vi "Configure Frequency Offset.vi"(0 "VISA resource name":refnum<visa-resource-name>, 1 "Multiplier (1)":i32=1, 3 "Divisor (1)":i32=1, 4 "Offset (0.0)":dbl format="%^.3g", 5 "error in (no error)":errorcluster, 6 "Channel (1)":i32=1, 7 "Start (300.0E+3)":dbl=300000.0 format="%^.1e", 9 "Stop (300.0E+3)":dbl=300000.0 format="%^.1g", 10 "External Frequency State (F: Disabled)":bool, 11 "Avoid Spurious (F: Off)":bool, 12 "Port (1)":i32=1, 13 "X Axis Frequency (0: Normal Frequency)":u16(ring) items=["Normal frequency", "Normal frequency + frequency of the external signal source", "Normal frequency - frequency of the external signal source", "Frequency of the external signal source - normal frequency", "Normal frequency", "Frequency for the source port for the specified measurement parameter", "Frequency for the receiver port for the specified measurement parameter"]) -> (14 "VISA resource name out":refnum<visa-resource-name>, 19 "error out":errorcluster)   [LabVIEW 2020, in "Agilent ENA Series.lvlib"]
doc: "Configures frequency offset parameters.\n\n<B>Note:</B>\nThis VI is not valid for E5061B/E5063A, E5080A and E5080B."
uses:
  <instrlib>/Agilent ENA Series/Agilent ENA Series.lvlib
panel:
  # "Note:\nThis VI is not supported by the E5061B/E5063A, E5080A and E5080B."
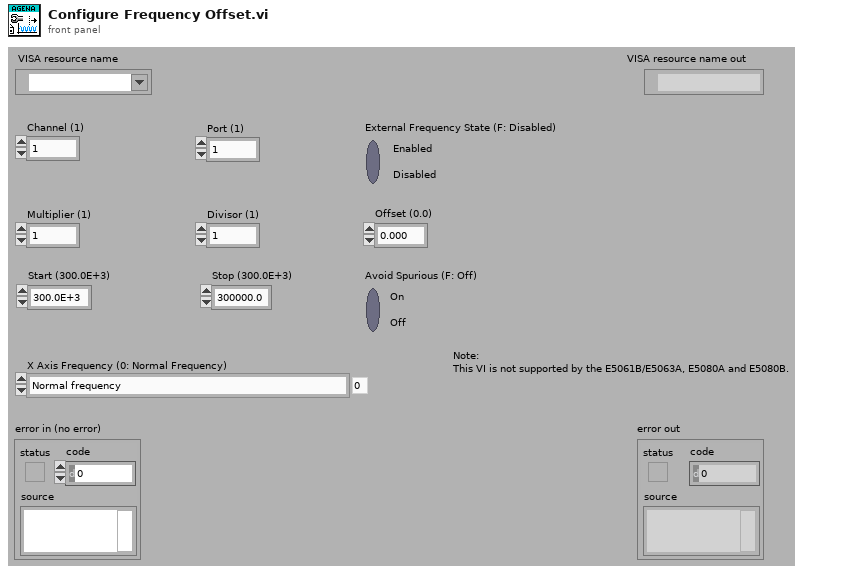
[diagram p1: front panel]
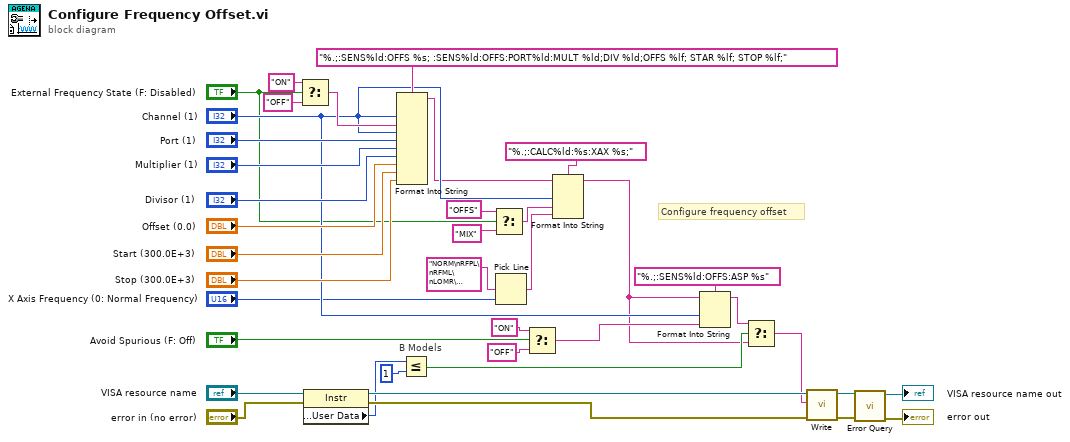
[diagram p0: block diagram]
diagram:
  # "Configure frequency offset"
  # "B Models"
  n1 = Select(t="ON", s="External Frequency State (F: Disabled)", f="OFF") -> (s? t:f=w36:string)
  n2 = property on="Property Node" class="Instr"(reference="VISA resource name", error in="error in (no error)") -> (reference out=w8:refnum<visa-resource-name>, error out=w7:errorcluster, "General Settings:User Data"=w5:u32)
  n3 = Format Into String(format string="%.;:SENS%ld:OFFS %s; :SENS%ld:OFFS:PORT%ld:MULT %ld;DIV %ld;OFFS %lf; STAR %lf; STOP %lf;", "Channel (1)", w36, "Channel (1)", "Port (1)", "Multiplier (1)", "Divisor (1)", "Offset (0.0)", "Start (300.0E+3)", "Stop (300.0E+3)") -> (resulting string=w2:string)  [unwired: 2 in, 1 out]
  n4 = Less Or Equal?(x=w5, y=u32 1) -> (x <= y?=w6:bool)
  n5 = Select(t="OFFS", s="External Frequency State (F: Disabled)", f="MIX") -> (s? t:f=w13:string)
  n6 = Pick Line(multi-line string="NORM\nRFPL\nRFML\nLOMR\nBASE\nSTIM\nRESP", line index="X Axis Frequency (0: Normal Frequency)") -> (output string=w16:string)  [unwired: 1 in]
  n7 = Select(t="ON", s="Avoid Spurious (F: Off)", f="OFF") -> (s? t:f=w20:string)
  n8 = Format Into String(format string="%.;:CALC%ld:%s:XAX %s;", initial string=w2, "Channel (1)", w13, w16) -> (resulting string=w3:string)  [unwired: 1 in, 1 out]
  n9 = Format Into String(format string="%.;:SENS%ld:OFFS:ASP %s", initial string=w3, "Channel (1)", w20) -> (resulting string=w11:string)  [unwired: 1 in, 1 out]
  n10 = Select(t=w11, s=w6, f=w3) -> (s? t:f=w1:string)
  n11 = call <instrlib>:"Write.vi"("error in (no error)"=w7, "String ()"=w1, "VISA resource name"=w8) -> ("error out"=w26:errorcluster, "VISA resource name out"=w27:refnum<visa-resource-name>)  [unwired: 6 in, 1 out]
  n12 = call <instrlib>:"Error Query.vi"("error in (no error)"=w26, "VISA resource name"=w27) -> ("error out"=→"error out":errorcluster, "VISA resource name out"=→"VISA resource name out":refnum<visa-resource-name>)  [unwired: 6 in, 2 out]
